vi "LP-AP filter.vi"(10 "Input":dbl) -> (0 "LP/AP":bool, 2 "Output":u16)   [LabVIEW 2013, in "ProcessorHelperFunctions.lvlib"]
uses:
  ProcessorHelperFunctions.lvlib
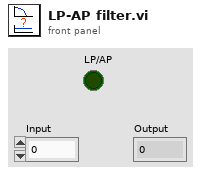
[diagram p1: front panel]
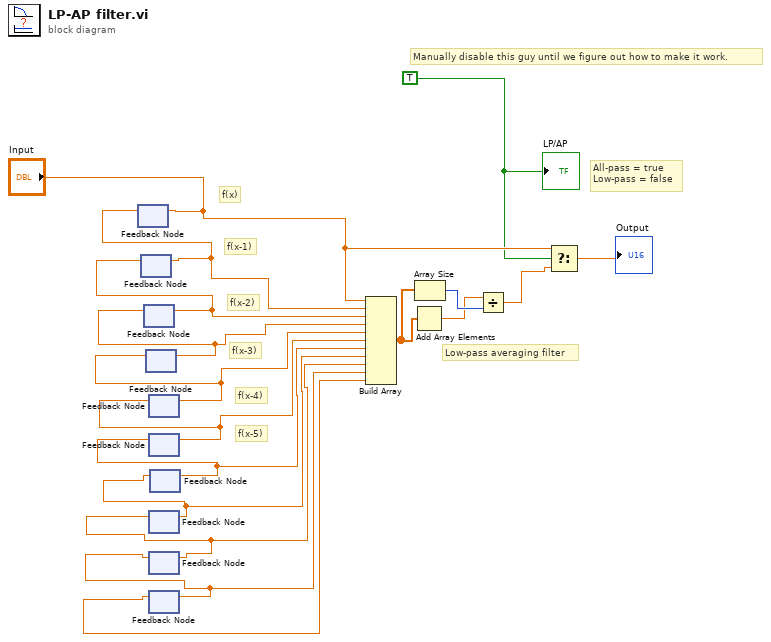
[diagram p0: block diagram]
diagram:
  w7 = TRUE
  # "Manually disable this guy until we figure out how to make it work."
  # "All-pass = true\nLow-pass = false"
  # "Low-pass averaging filter"
  # "f(x-5)"
  # "f(x-4)"
  # "f(x-3)"
  # "f(x-2)"
  # "f(x-1)"
  # "f(x)"
  n1 = feedback-in #1("Input") -> ()
  n2 = feedback #1() -> (w10:dbl)  [unwired: 1 in]
  n3 = feedback #2() -> (w17:dbl)  [unwired: 1 in]
  n4 = feedback-in #2(w10) -> ()
  n5 = feedback #3() -> (w16:dbl)  [unwired: 1 in]
  n6 = feedback-in #3(w17) -> ()
  n7 = feedback #4() -> (w15:dbl)  [unwired: 1 in]
  n8 = feedback-in #4(w16) -> ()
  n9 = feedback #5() -> (w6:dbl)  [unwired: 1 in]
  n10 = feedback-in #5(w15) -> ()
  n11 = feedback #6() -> (w5:dbl)  [unwired: 1 in]
  n12 = feedback-in #6(w6) -> ()
  n13 = feedback #7() -> (w3:dbl)  [unwired: 1 in]
  n14 = feedback #8() -> (w2:dbl)  [unwired: 1 in]
  n15 = feedback-in #8(w3) -> ()
  n16 = feedback #9() -> (w1:dbl)  [unwired: 1 in]
  n17 = feedback-in #9(w2) -> ()
  n18 = feedback #10() -> (w4:dbl)  [unwired: 1 in]
  n19 = feedback-in #7(w4) -> ()
  n20 = feedback-in #10(w5) -> ()
  n21 = Build Array("Input", w10, w17, w16, w15, w6, w5, w4, w3, w2, w1) -> (w14:dbl[])
  n22 = Add Array Elements(numeric array=w14) -> (sum=w12:dbl)
  n23 = Array Size(array=w14) -> (size(s)=w13:i32)
  n24 = Divide(x=w12, y=w13) -> (x/y=w11:dbl)
  n25 = Select(t="Input", s=w7, f=w11) -> (s? t:f=→"Output":dbl)
  "LP/AP" <- w7
